vi "E441X_PM_Session_Info.vi"(0 "VISA session":refnum<visa-resource-name>, 1 "Sensor A (0:None)":i32(ring) items=["None", "8480", "E Series", "E9320"], 2 "Operation":i32(ring) items=["Set", "Get"], 7 "Instrument Number (16)":i32, 11 "error in (no error)":errorcluster {"code" format="%.0x"}, 12 "Sensor B (0:None)":i32(ring) items=["None", "8480", "E Series", "E9320"]) -> (3 "Sensor A (0: None)":i32(ring) items=["None", "8480", "E Series", "E9320"], 4 "dup VISA session":refnum<visa-resource-name>, 8 "Instrument Number":i32, 10 "Channels":i32, 14 "Sensor B (0: None)":i32(ring) items=["None", "8480", "E Series", "E9320"], 15 "error out":errorcluster {"code" format="%.0x"})   [LabVIEW 2015]
doc: "This VI sets/gets the session info."
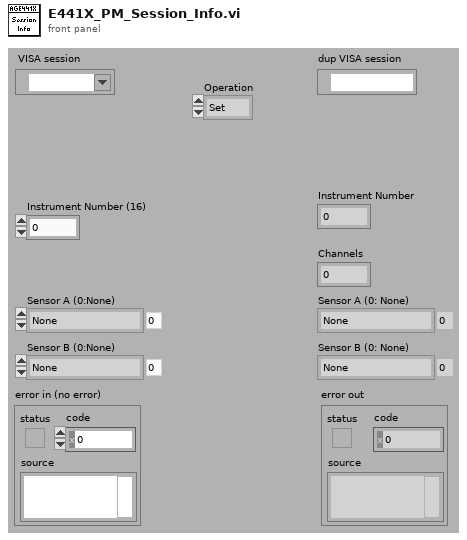
[diagram p1: front panel]
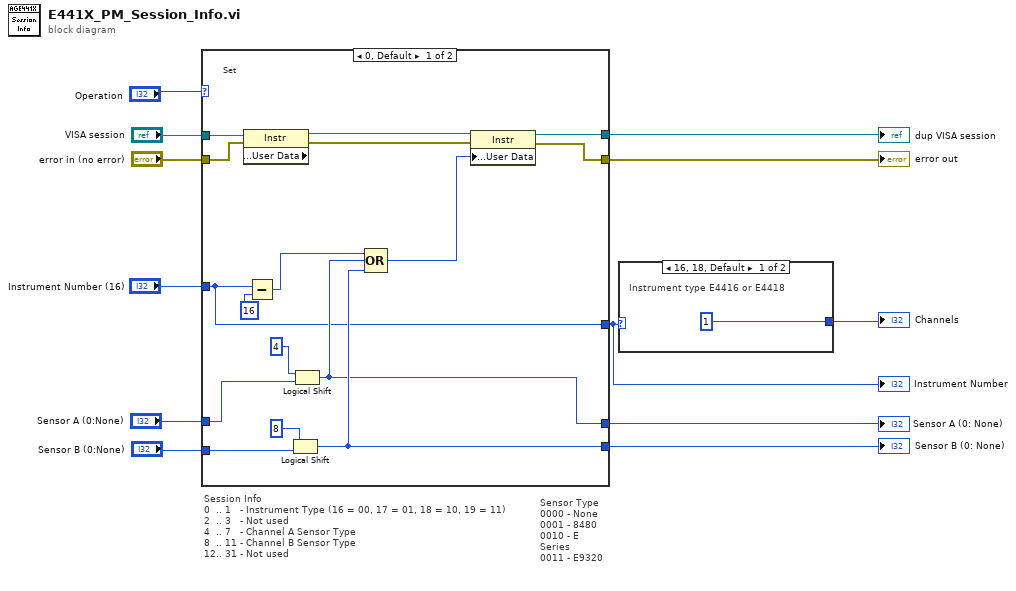
[diagram p0: block diagram]
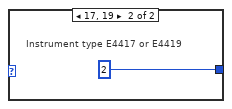
[diagram p2: hidden frame]
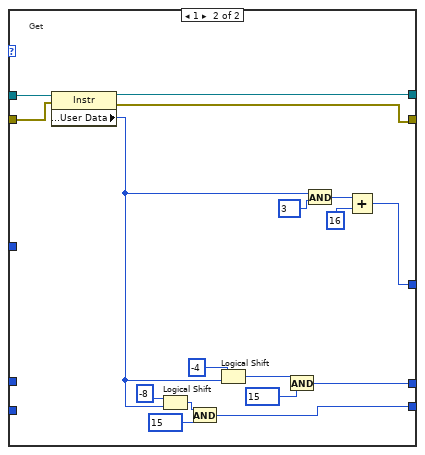
[diagram p3: hidden frame]
diagram:
  # "Sensor Type\n0000 - None\n0001 - 8480\n0010 - E Series\n0011 - E9320"
  # "Session Info\n0  .. 1   - Instrument Type (16 = 00, 17 = 01, 18 = 10, 19 = 11)\n2  .. 3   - Not used\n4  .. 7   - Channel A Sensor Type\n8  .. 11 - Channel B Sensor Type\n12.. 31 - Not used"
  n1 = case shown="0, Default" "Operation" {
    tunnel: "VISA session" -> [w16 w45]
    tunnel: "error in (no error)" -> [w15 w44]
    tunnel: "Instrument Number (16)" -> [w18 _]
    tunnel: "Sensor A (0:None)" -> [w17 _]
    tunnel: "Sensor B (0:None)" -> [w25 _]
    tunnel: [w22 w42] -> w6
    tunnel: [w21 w43] -> w5
    tunnel: [w20 w33] -> w4
    tunnel: [w19 w32] -> w3
    tunnel: [w18 w38] -> w1
    frame 0, Default {
      # "Set"
      n2 = property class="Instr" props=["General Settings:User Data"](reference=w16, error in=w15) -> (reference out=w14:refnum<visa-resource-name>, error out=w13:errorcluster)  [unwired: 1 out]
      n3 = Subtract(x=w18, y=16) -> (x-y=w27:i32)
      n4 = Logical Shift(y=u8 8, x=w25) -> (x << y=w20:i32)
      n5 = Logical Shift(y=u8 4, x=w17) -> (x << y=w19:i32)
      n6 = Compound Arithmetic op=OR(w27, w19, w20) -> (w23:i32)
      n7 = property class="Instr"(reference=w14, error in=w13, "General Settings:User Data"=w23) -> (reference out=w22:refnum<visa-resource-name>, error out=w21:errorcluster)
    }
    frame 1 {
      # "Get"
      n8 = property class="Instr"(reference=w45, error in=w44) -> (reference out=w42:refnum<visa-resource-name>, error out=w43:errorcluster, "General Settings:User Data"=w30:u32)
      n9 = Logical Shift(y=-8, x=w30) -> (x << y=w34:u32)
      n10 = And(x=w34, y=15) -> (x .and. y?=w33:u32)
      n11 = Logical Shift(y=-4, x=w30) -> (x << y=w29:u32)
      n12 = And(x=w29, y=15) -> (x .and. y?=w32:u32)
      n13 = And(x=w30, y=3) -> (x .and. y?=w40:u32)
      n14 = Add(x=w40, y=u32 16) -> (x+y=w38:u32)
    }
  }
  "error out" <- w5
  "dup VISA session" <- w6
  "Instrument Number" <- w1
  "Sensor B (0: None)" <- w4
  "Sensor A (0: None)" <- w3
  n15 = case shown="16, 18, Default" w1 {
    tunnel: [1 ("Channels") 2 ("Channels")] -> w2
    frame 16, 18, Default {
      # "Instrument type E4416 or E4418"
    }
    frame 17, 19 {
      # "Instrument type E4417 or E4419"
    }
  }
  "Channels" <- w2
